vi "emi_Close Application.vi"(11 "error in (no error)":errorcluster) -> (15 "error out":errorcluster)   [LabVIEW 2011]
doc: "Close the application. \n\nThis VI disregards Error in, and does not give error out. \n\nIf application it closes teh exe.\nIf runnig in the development enviroment, it ends teh program, leving the VIs open"
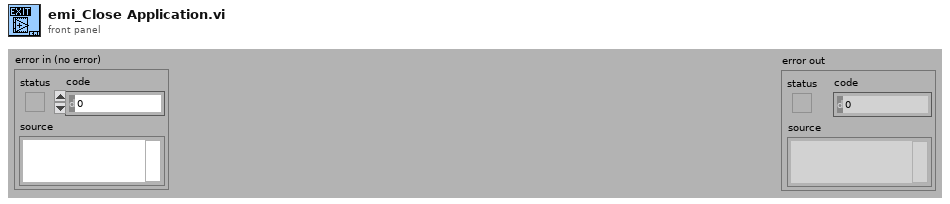
[diagram p1: front panel]
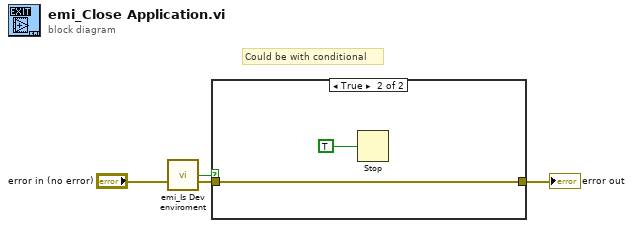
[diagram p0: block diagram]
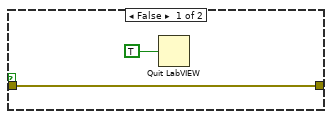
[diagram p2: hidden frame]
diagram:
  # "Could be with conditional"
  n1 = call "emi_Is Dev enviroment.vi"("error in (no error)"="error in (no error)") -> ("Dev System?"=w3:bool, "error out"=w1:errorcluster)  [unwired: 13 in]
  n2 = case shown="True" w3 {
    tunnel: [w5 w8] -> w4
    tunnel: w1 -> [w5 w8]
    frame False {
      n3 = Quit LabVIEW(quit? (T)=TRUE) -> ()
    }
    frame True {
      n4 = Stop(stop? (T)=TRUE) -> ()
    }
  }
  "error out" <- w4
